vi "FindFormatsInString.vi"(9 "Font":T2, 10 "Color":u32, 11 "StringsIn":string[](array[string])) -> (1 "StringsOut":string[](array[string]), 3 "Formats":T1(array[cluster]))   [LabVIEW 2014, in "Graphics.lvclass"]
uses:
  <resource>/Framework/Providers/Open_GDS/UML/Graphics_class/Graphics.lvclass
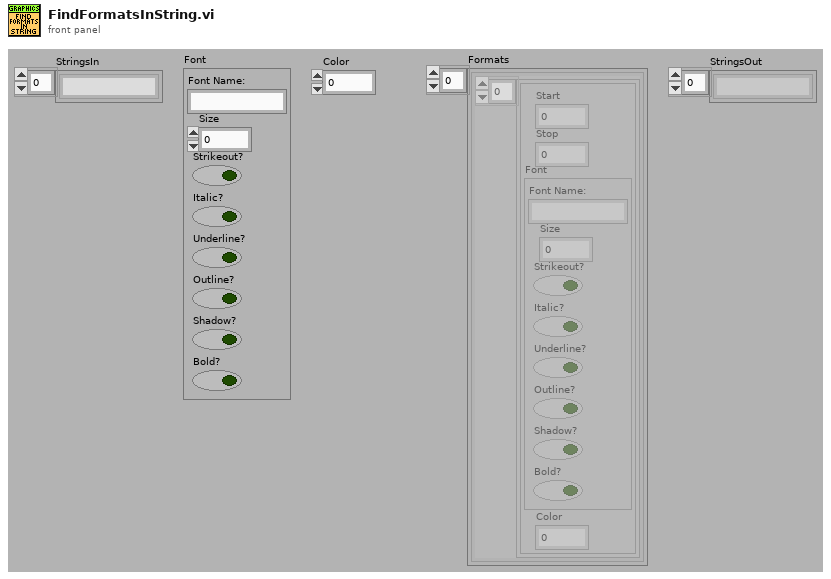
[diagram p1: front panel]
types:
  T1 = cluster{cluster{"Start":i32, "Stop":i32, "Font":cluster{"Font Name:":string, "Size":i16, "Strikeout?":bool, "Italic?":bool, "Underline?":bool, "Outline?":bool, "Shadow?":bool, "Bold?":bool}, "Color":u32}[]}[]
  T2 = cluster{"Font Name:":string, "Size":i16, "Strikeout?":bool, "Italic?":bool, "Underline?":bool, "Outline?":bool, "Shadow?":bool, "Bold?":bool}
  T3 = cluster{"Start":i32, "Stop":i32, "Font":cluster{"Font Name:":string, "Size":i16, "Strikeout?":bool, "Italic?":bool, "Underline?":bool, "Outline?":bool, "Shadow?":bool, "Bold?":bool}, "Color":u32}
  T4 = cluster{"Start":i32, "Stop":i32, "Font":cluster{"Font Name:":string, "Size":i16, "Strikeout?":bool, "Italic?":bool, "Underline?":bool, "Outline?":bool, "Shadow?":bool, "Bold?":bool}, "Color":u32}[]
  T5 = cluster{cluster{"Start":i32, "Stop":i32, "Font":cluster{"Font Name:":string, "Size":i16, "Strikeout?":bool, "Italic?":bool, "Underline?":bool, "Outline?":bool, "Shadow?":bool, "Bold?":bool}, "Color":u32}[]}
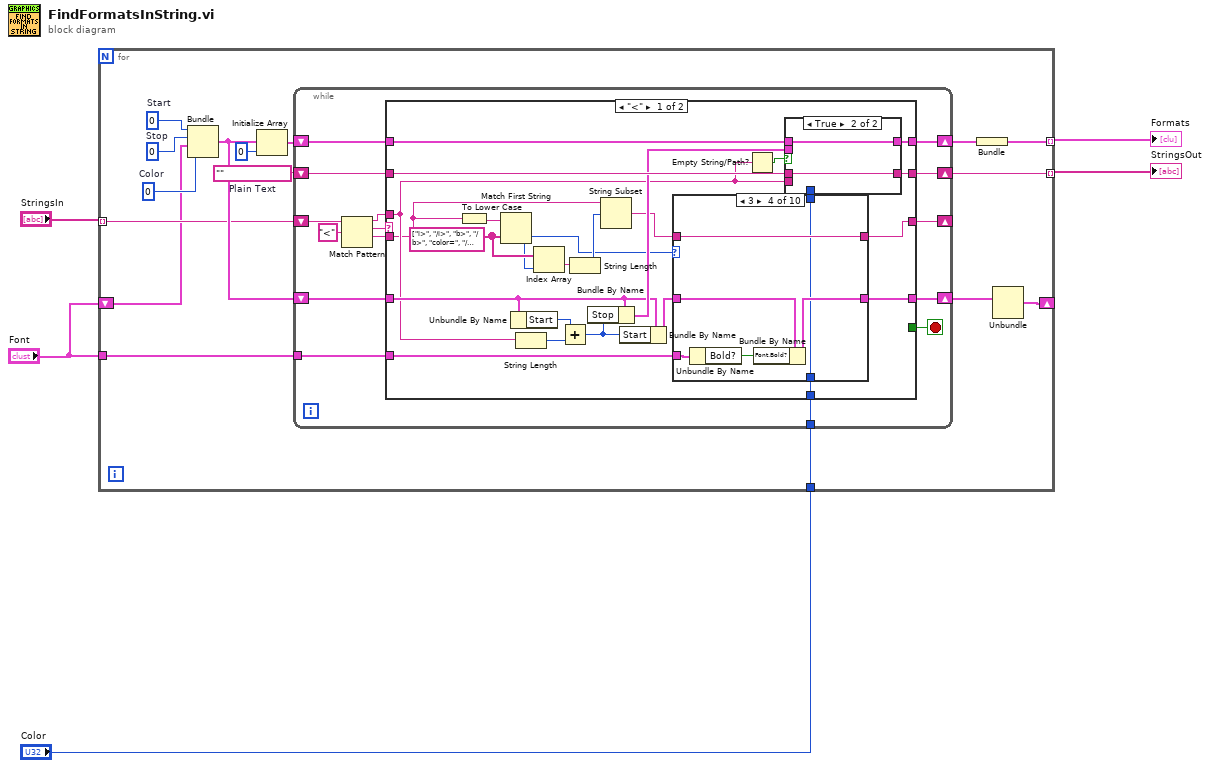
[diagram p0: block diagram]
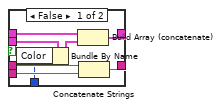
[diagram p2: hidden frame]
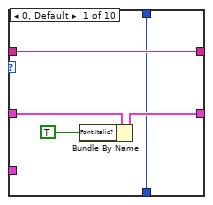
[diagram p3: hidden frame]
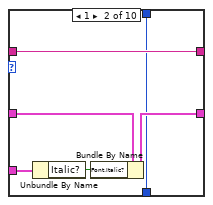
[diagram p4: hidden frame]
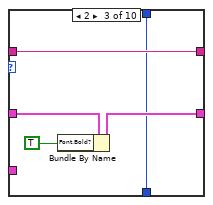
[diagram p5: hidden frame]
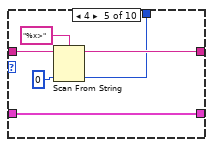
[diagram p6: hidden frame]
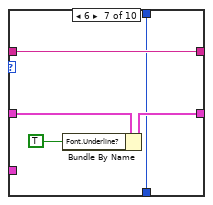
[diagram p8: hidden frame]
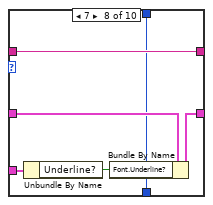
[diagram p9: hidden frame]
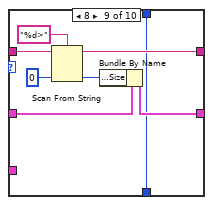
[diagram p10: hidden frame]
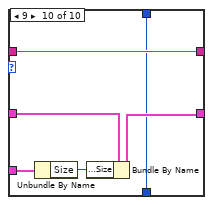
[diagram p11: hidden frame]
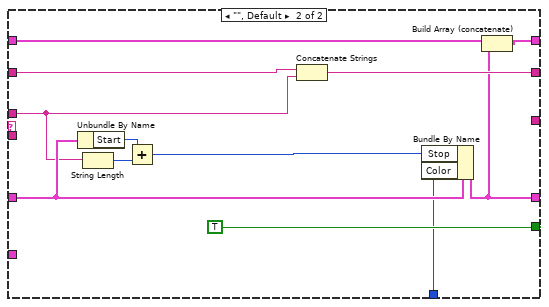
[diagram p12: hidden frame]
diagram:
  n1 = for {
    tunnel: "StringsIn" -> [w15] mode=indexing
    tunnel: [w14] -> w3 mode=indexing
    tunnel: [w12] -> w2 mode=indexing
    tunnel: "Color" -> [w10]
    tunnel: "Font" -> [w8]
    shift-right: [w6] -> _
    shift-left: "Font" -> [w7]
    w11 = u32 0  # Color
    w17 = ""  # Plain Text
    w20 = 0  # Stop
    w21 = 0  # Start
    n2 = Bundle("Start"=w21, "Stop"=w20, "Font"=w7, "Color"=w11) -> (w18:T3)  [unwired: 1 out]
    n3 = Initialize Array(w18, 0 ("dimension size")) -> (w19:T4)
    n4 = while {
      shift-right: [w28] -> w13
      shift-left: w19 -> [w31]
      shift-right: [w30] -> _
      shift-left: w15 -> [w36]
      shift-right: [w27] -> w9
      shift-left: w18 -> [w29]
      tunnel: w8 -> [w25]
      shift-right: [w23] -> w14
      shift-left: w17 -> [w24]
      tunnel: w10 -> [w22]
      stop <- w26 stop-if-true
      n5 = Match Pattern(string=w36, regular expression="<") -> (before substring=w33:string, match substring=w34:string, after substring=w32:string)  [unwired: 2 out]
      n6 = case shown="\"<\"" w34 {
        tunnel: w33 -> [w47 w129]
        tunnel: w32 -> [w41 _]
        tunnel: w31 -> [w55 w135]
        tunnel: [w58 _] -> w30
        tunnel: w29 -> [w49 w130]
        tunnel: [w54 w134] -> w28
        tunnel: [w60 w133] -> w27
        tunnel: [_ TRUE] -> w26
        tunnel: w25 -> [w59 _]
        tunnel: w24 -> [w57 w136]
        tunnel: [w56 w137] -> w23
        tunnel: w22 -> [w37 w127]
        frame "<" {
          w43 = string[] ["i>", "/i>", "b>", "/b>", "color=", "/color>", "u>", "/u>", "size=", "/size>"] ("string array")
          n7 = To Lower Case(string=w41) -> (all lower case string=w42:string)
          n8 = Match First String(2:w43, 3:w42) -> (0:w39:i32)  [unwired: 1 out]
          n9 = Unbundle By Name(w49) -> ("Start"=w52:i32)
          n10 = String Length(string=w47) -> (length=w53:i32)
          n11 = Index Array(array=w43, index=w39) -> (element=w44:string)
          n12 = Add(x=w52, y=w53) -> (x+y=w50:i32)
          n13 = String Length(string=w44) -> (length=w45:i32)
          n14 = Bundle By Name(cluster=w49, "Stop"=w50) -> (w51:T3)
          n15 = String Subset(string=w41, offset (0)=w45) -> (substring=w40:string)  [unwired: 1 in]
          n16 = Bundle By Name(cluster=w49, "Start"=w50) -> (w48:T3)
          n17 = case shown="3" w39 {
            tunnel: w48 -> [w73 w80 w84 w91 w93 w100 w104 w111 w119 w125]
            tunnel: [w75 w81 w86 w92 w93 w100 w106 w112 w120 w126] -> w60
            tunnel: w59 -> [_ w79 _ w90 _ _ _ w110 _ w123]
            tunnel: w40 -> [w72 w77 w83 w88 w98 w101 w103 w108 w118 w124]
            tunnel: [w72 w77 w83 w88 w95 w101 w103 w108 w114 w124] -> w58
            tunnel: [w71 w76 w82 w87 w94 w99 w102 w107 w113 w121] -> w38
            tunnel: w37 -> [w71 w76 w82 w87 _ w99 w102 w107 w113 w121]
            frame 0, Default {
              n18 = Bundle By Name(cluster=w73, "Font.Italic?"=TRUE ("Default Properties.Italic?")) -> (w75:T3)
            }
            frame 1 {
              n19 = Unbundle By Name(w79) -> ("Italic?"=w78:bool)
              n20 = Bundle By Name(cluster=w80, "Font.Italic?"=w78) -> (w81:T3)
            }
            frame 2 {
              n21 = Bundle By Name(cluster=w84, "Font.Bold?"=TRUE ("Default Properties.Italic?")) -> (w86:T3)
            }
            frame 3 {
              n22 = Unbundle By Name(w90) -> ("Bold?"=w89:bool)
              n23 = Bundle By Name(cluster=w91, "Font.Bold?"=w89) -> (w92:T3)
            }
            frame 4 {
              n24 = Scan From String(format string="%x>", input string=w98, default 1=u32 0 ("default value 1")) -> (remaining string=w95:string, output 1=w94:u32)  [unwired: 2 in, 2 out]
            }
            frame 5 {
            }
            frame 6 {
              n25 = Bundle By Name(cluster=w104, "Font.Underline?"=TRUE ("Default Properties.Italic?")) -> (w106:T3)
            }
            frame 7 {
              n26 = Unbundle By Name(w110) -> ("Underline?"=w109:bool)
              n27 = Bundle By Name(cluster=w111, "Font.Underline?"=w109) -> (w112:T3)
            }
            frame 8 {
              n28 = Scan From String(format string="%d>", input string=w118, default 1=i16 0 ("default value 1")) -> (remaining string=w114:string, output 1=w116:i16)  [unwired: 2 in, 2 out]
              n29 = Bundle By Name(cluster=w119, "Font.Size"=w116) -> (w120:T3)
            }
            frame 9 {
              n30 = Unbundle By Name(w123) -> ("Size"=w122:i16)
              n31 = Bundle By Name(cluster=w125, "Font.Size"=w122) -> (w126:T3)
            }
          }
          n32 = Empty String/Path?(string/path=w47) -> (empty?=w46:bool)
          n33 = case shown="True" w46 {
            tunnel: w57 -> [w68 w69]
            tunnel: [w67 w69] -> w56
            tunnel: w55 -> [w66 w70]
            tunnel: [w65 w70] -> w54
            tunnel: w51 -> [w63 _]
            tunnel: w47 -> [w64 _]
            tunnel: w38 -> [w61 _]
            frame False {
              n34 = Bundle By Name(cluster=w63, "Color"=w61) -> (w62:T3)
              n35 = Build Array (concatenate)(w66, w62) -> (w65:T4)
              n36 = Concatenate Strings(w68, w64) -> (w67:string)
            }
            frame True {
            }
          }
        }
        frame "", Default {
          n37 = Unbundle By Name(w130) -> ("Start"=w131:i32)
          n38 = String Length(string=w129) -> (length=w132:i32)
          n39 = Add(x=w131, y=w132) -> (x+y=w128:i32)
          n40 = Concatenate Strings(w136, w129) -> (w137:string)
          n41 = Bundle By Name(cluster=w130, "Stop"=w128, "Color"=w127) -> (w133:T3)
          n42 = Build Array (concatenate)(w135, w133) -> (w134:T4)
        }
      }
    }
    n43 = Bundle(w13) -> (w12:T5)  [unwired: 1 in]
    n44 = Unbundle(w9) -> ("Font"=w6:T2)  [unwired: 3 out]
  }
  "StringsOut" <- w3
  "Formats" <- w2
